vi "CRYReCalc Arith X-combi.vi"(6 "X-axis Combination":u16, 7 "Curve_In":cluster{"x":dbl, "y":dbl, "z":dbl}[](array[cluster]) {"z" format="%.2f"; "y" format="%.2f"; "x" format="%.2f"}, 8 "Curve A":T1={"Name"="", "Curve"=[], "X data"=1, "Y data"=1, "Z data"=1, "X axis"=0, "Y axis"=1, "Z axis"=1, "X unit"="Hz", "Y unit"="", "Z unit"="deg.", "X dB ref"=1.0, "Y dB ref"=1.0, "Z dB ref"=1.0, "single val"=FALSE, "protected"=FALSE, "display X"=TRUE, "display Y"=TRUE, "display Z"=TRUE, "Test Info"="", "Step No."=0, "Plot Settings"={"Color"=0, "Interpolation"=0, "Point Style"=0, "Line Style"=0, "Point Color"=0, "Line Width"=0, "Bar Plot Style"=0, "Fill To"=0}, "AutoProtect"=FALSE} {"Z data" items=["dB", "Lin"]; "X data" items=["dB", "Lin"]; "Y data" items=["dB", "Lin"]; "Z dB ref" format="%.1f"; "Z axis" items=["Log", "Lin"]; "X dB ref" format="%.1f"; "X axis" items=["Log", "Lin"]; "Y axis" items=["Log", "Lin"]; "Y dB ref" format="%.1f"; "Curve"."z" format="%.2f"; "Curve"."y" format="%.2f"; "Curve"."x" format="%.2f"}, 11 "Curve B":T1={"Name"="", "Curve"=[], "X data"=1, "Y data"=1, "Z data"=1, "X axis"=0, "Y axis"=1, "Z axis"=1, "X unit"="Hz", "Y unit"="", "Z unit"="deg.", "X dB ref"=1.0, "Y dB ref"=1.0, "Z dB ref"=1.0, "single val"=FALSE, "protected"=FALSE, "display X"=TRUE, "display Y"=TRUE, "display Z"=TRUE, "Test Info"="", "Step No."=0, "Plot Settings"={"Color"=0, "Interpolation"=0, "Point Style"=0, "Line Style"=0, "Point Color"=0, "Line Width"=0, "Bar Plot Style"=0, "Fill To"=0}, "AutoProtect"=FALSE} {"Z data" items=["dB", "Lin"]; "X data" items=["dB", "Lin"]; "Y data" items=["dB", "Lin"]; "Z dB ref" format="%.1f"; "Z axis" items=["Log", "Lin"]; "X dB ref" format="%.1f"; "X axis" items=["Log", "Lin"]; "Y axis" items=["Log", "Lin"]; "Y dB ref" format="%.1f"; "Curve"."z" format="%.2f"; "Curve"."y" format="%.2f"; "Curve"."x" format="%.2f"}) -> (1 "Curve_Out":cluster{"x":dbl, "y":dbl, "z":dbl}[](array[cluster]))   [LabVIEW 2013]
uses:
  Typedef Control/CRYData Cluster.ctl
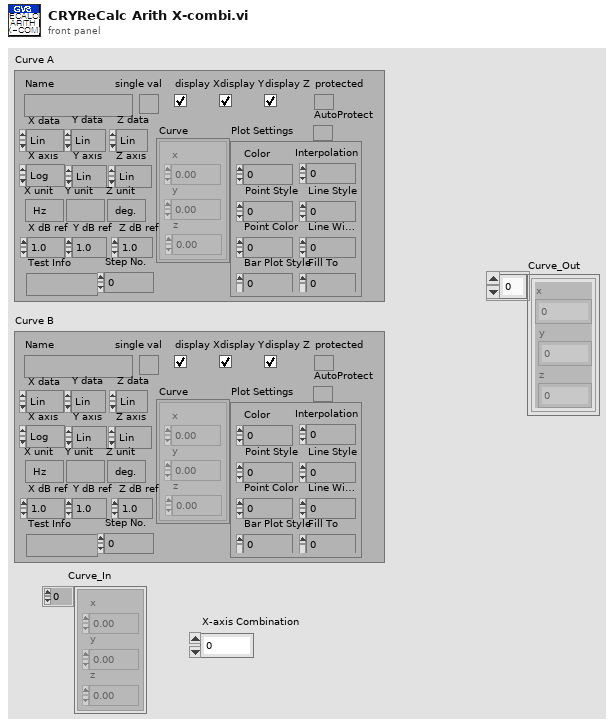
[diagram p1: front panel]
types:
  T1 = typedef "CRYData Cluster.ctl" = cluster{"Name":string, "Curve":cluster{"x":dbl, "y":dbl, "z":dbl}[], "X data":u16, "Y data":u16, "Z data":u16, "X axis":u16, "Y axis":u16, "Z axis":u16, "X unit":string, "Y unit":string, "Z unit":string, "X dB ref":dbl, "Y dB ref":dbl, "Z dB ref":dbl, "single val":bool, "protected":bool, "display X":bool, "display Y":bool, "display Z":bool, "Test Info":string, "Step No.":i32, "Plot Settings":cluster{"Color":u32, "Interpolation":u8, "Point Style":u8, "Line Style":u8, "Point Color":u32, "Line Width":u8, "Bar Plot Style":u8, "Fill To":i16}, "AutoProtect":bool}
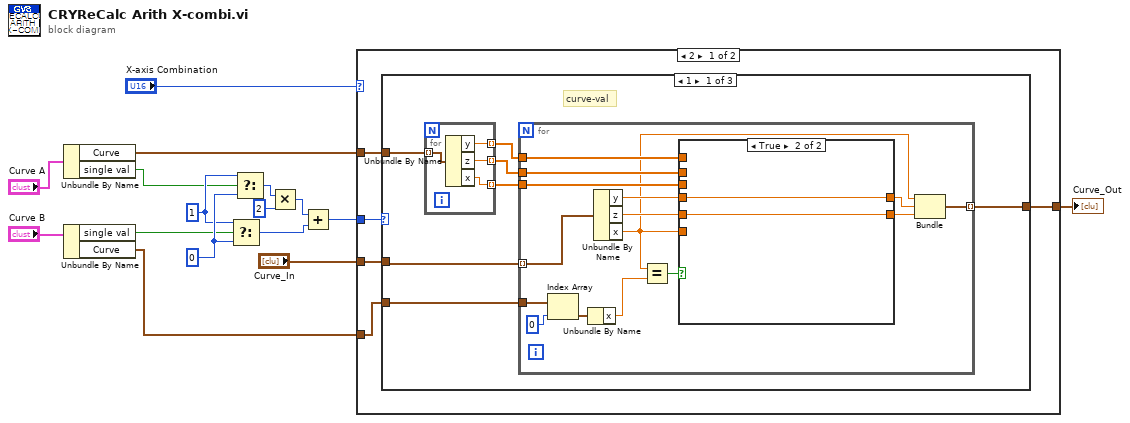
[diagram p0: block diagram]
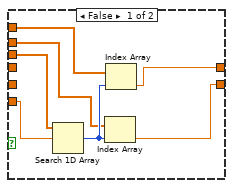
[diagram p2: hidden frame]
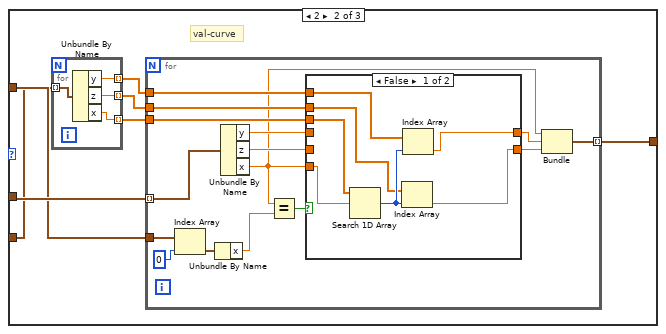
[diagram p3: hidden frame]
diagram:
  w14 = 1
  w15 = 0
  n1 = Unbundle By Name("Curve A") -> ("Curve"=w3:cluster{"x":dbl, "y":dbl, "z":dbl}[], "single val"=w9:bool)
  n2 = Unbundle By Name("Curve B") -> ("single val"=w8:bool, "Curve"=w2:cluster{"x":dbl, "y":dbl, "z":dbl}[])
  n3 = Select(t=w14, s=w8, f=w15) -> (s? t:f=w5:i32)
  n4 = Select(t=w14, s=w9, f=w15) -> (s? t:f=w7:i32)
  n5 = Multiply(x=w7, y=2) -> (x*y=w6:i32)
  n6 = Add(x=w6, y=w5) -> (x+y=w4:i32)
  n7 = case shown="2" "X-axis Combination" {
    tunnel: "Curve_In" -> [w21 w93]
    tunnel: [w20 w93] -> w1
    tunnel: w4 -> [w19 _]
    tunnel: w3 -> [w17 _]
    tunnel: w2 -> [w18 _]
    frame 2 {
      n8 = case shown="1" w19 {
        tunnel: w21 -> [w27 w63 w92]
        tunnel: [w22 w57 w92] -> w20
        tunnel: w18 -> [w28 w58 _]
        tunnel: w17 -> [w26 w59 _]
        frame 1 {
          # "curve-val"
          n9 = for {
            tunnel: w26 -> [w32] mode=indexing
            tunnel: [w31] -> w25 mode=indexing
            tunnel: [w30] -> w24 mode=indexing
            tunnel: [w29] -> w23 mode=indexing
            n10 = Unbundle By Name(w32) -> ("y"=w29:dbl, "z"=w30:dbl, "x"=w31:dbl)
          }
          n11 = for {
            tunnel: [w43] -> w22 mode=indexing
            tunnel: w28 -> [w40]
            tunnel: w27 -> [w39] mode=indexing
            tunnel: w25 -> [w36]
            tunnel: w24 -> [w35]
            tunnel: w23 -> [w34]
            n12 = Index Array(array=w40, index=0) -> (element=w38:cluster{"x":dbl, "y":dbl, "z":dbl})
            n13 = Unbundle By Name(w38) -> ("x"=w37:dbl)
            n14 = Unbundle By Name(w39) -> ("y"=w41:dbl, "z"=w42:dbl, "x"=w33:dbl)
            n15 = Equal?(x=w33, y=w37) -> (x = y?=w46:bool)
            n16 = case shown="True" w46 {
              tunnel: w41 -> [_ w56]
              tunnel: w42 -> [_ w55]
              tunnel: [w50 w56] -> w45
              tunnel: [w49 w55] -> w44
              tunnel: w36 -> [w54 _]
              tunnel: w35 -> [w52 _]
              tunnel: w34 -> [w51 _]
              tunnel: w33 -> [w48 _]
              frame False {
                n17 = Search 1D Array(1D array=w54, element=w48) -> (index of element=w53:i32)  [unwired: 1 out]
                n18 = Index Array(array=w52, index=w53) -> (element=w49:dbl)
                n19 = Index Array(array=w51, index=w53) -> (element=w50:dbl)
              }
              frame True {
              }
            }
            n20 = Bundle("x"=w33, "y"=w45, "z"=w44) -> (w43:cluster{"x":dbl, "y":dbl, "z":dbl})  [unwired: 1 in]
          }
        }
        frame 2 {
          # "val-curve"
          n21 = for {
            tunnel: w58 -> [w67] mode=indexing
            tunnel: [w66] -> w62 mode=indexing
            tunnel: [w65] -> w61 mode=indexing
            tunnel: [w64] -> w60 mode=indexing
            n22 = Unbundle By Name(w67) -> ("y"=w64:dbl, "z"=w65:dbl, "x"=w66:dbl)
          }
          n23 = for {
            tunnel: [w78] -> w57 mode=indexing
            tunnel: w59 -> [w75]
            tunnel: w63 -> [w74] mode=indexing
            tunnel: w62 -> [w71]
            tunnel: w61 -> [w70]
            tunnel: w60 -> [w69]
            n24 = Index Array(array=w75, index=0) -> (element=w73:cluster{"x":dbl, "y":dbl, "z":dbl})
            n25 = Unbundle By Name(w73) -> ("x"=w72:dbl)
            n26 = Unbundle By Name(w74) -> ("y"=w76:dbl, "z"=w77:dbl, "x"=w68:dbl)
            n27 = Equal?(x=w68, y=w72) -> (x = y?=w81:bool)
            n28 = case shown="False" w81 {
              tunnel: w76 -> [_ w91]
              tunnel: w77 -> [_ w90]
              tunnel: [w85 w91] -> w80
              tunnel: [w84 w90] -> w79
              tunnel: w71 -> [w89 _]
              tunnel: w70 -> [w87 _]
              tunnel: w69 -> [w86 _]
              tunnel: w68 -> [w83 _]
              frame False {
                n29 = Search 1D Array(1D array=w89, element=w83) -> (index of element=w88:i32)  [unwired: 1 out]
                n30 = Index Array(array=w87, index=w88) -> (element=w84:dbl)
                n31 = Index Array(array=w86, index=w88) -> (element=w85:dbl)
              }
              frame True {
              }
            }
            n32 = Bundle("x"=w68, "y"=w80, "z"=w79) -> (w78:cluster{"x":dbl, "y":dbl, "z":dbl})  [unwired: 1 in]
          }
        }
        frame 0, 3, Default {
        }
      }
    }
    frame 0, 1, Default {
    }
  }
  "Curve_Out" <- w1
